vi "运维调试_五参数.vi"() -> ()   [LabVIEW 2016, in "斯坦道仪器.lvlib"]
uses:
  <vilib>/Utility/miscctls.llb/LVPointTypeDef.ctl
  PLC/PLC.lvlib
panel:
  in  "打开串口":bool
  in  "释放串口":bool
  in  "手动通电":bool
  out "多参数横条运行状态":T1(xcontrol)
  in  "数据区":i32(listbox)
  in  "探头选择":u16(ring)=9 items=["氨氮"=3, "水温"=9, "pH值"=10, "溶解氧"=11, "电导率"=12, "浊度"=13, "叶绿素a"=14, "藻密度"=15, "蓝绿藻"=16, "氧化还原电位"=17, "溶解氧%"=18, "盐度"=19]
  in  "测量数据区读取":bool
  in  "测量数据区":i32(listbox)
  in  "状态告警区读取":bool
  in  "状态告警区":i32(listbox)
  in  "自动校准":bool
  in  "读取KB":bool
  in  "写入KB":bool
  out "B":dbl caption="校准值B:"
  out "K":dbl caption="校准值K:"
  in  "校准区探头选择":u16(ring)=9 items=["氨氮"=3, "水温"=9, "pH值"=10, "溶解氧"=11, "电导率"=12, "浊度"=13, "叶绿素a"=14, "藻密度"=15, "蓝绿藻"=16, "氧化还原电位"=17, "溶解氧%"=18, "盐度"=19]
  in  "停止测量(单探)":bool
  in  "启动测量(单探)":bool
  in  "控制命令区探头选择":u16(ring)=9 items=["氨氮"=3, "水温"=9, "pH值"=10, "溶解氧"=11, "电导率"=12, "浊度"=13, "叶绿素a"=14, "藻密度"=15, "蓝绿藻"=16, "氧化还原电位"=17, "溶解氧%"=18, "盐度"=19]
  in  "同步时间":bool
  in  "初始化(清洗)":bool
  in  "停止测量(全部)":bool
  in  "启动测量(全部)":bool
  in  "关键参数区读取":bool
  in  "关键参数区":i32(listbox)
  in  "传感器参数读取":bool
  in  "传感器区":i32(listbox)
  in  "返回":bool
  in  "设置":bool
  out "运行状态":string
  out "开机状态":bool
  in  "停止":bool
  in  "手动启动":bool
  out "集成报警信息":string
  # "控制命令区"
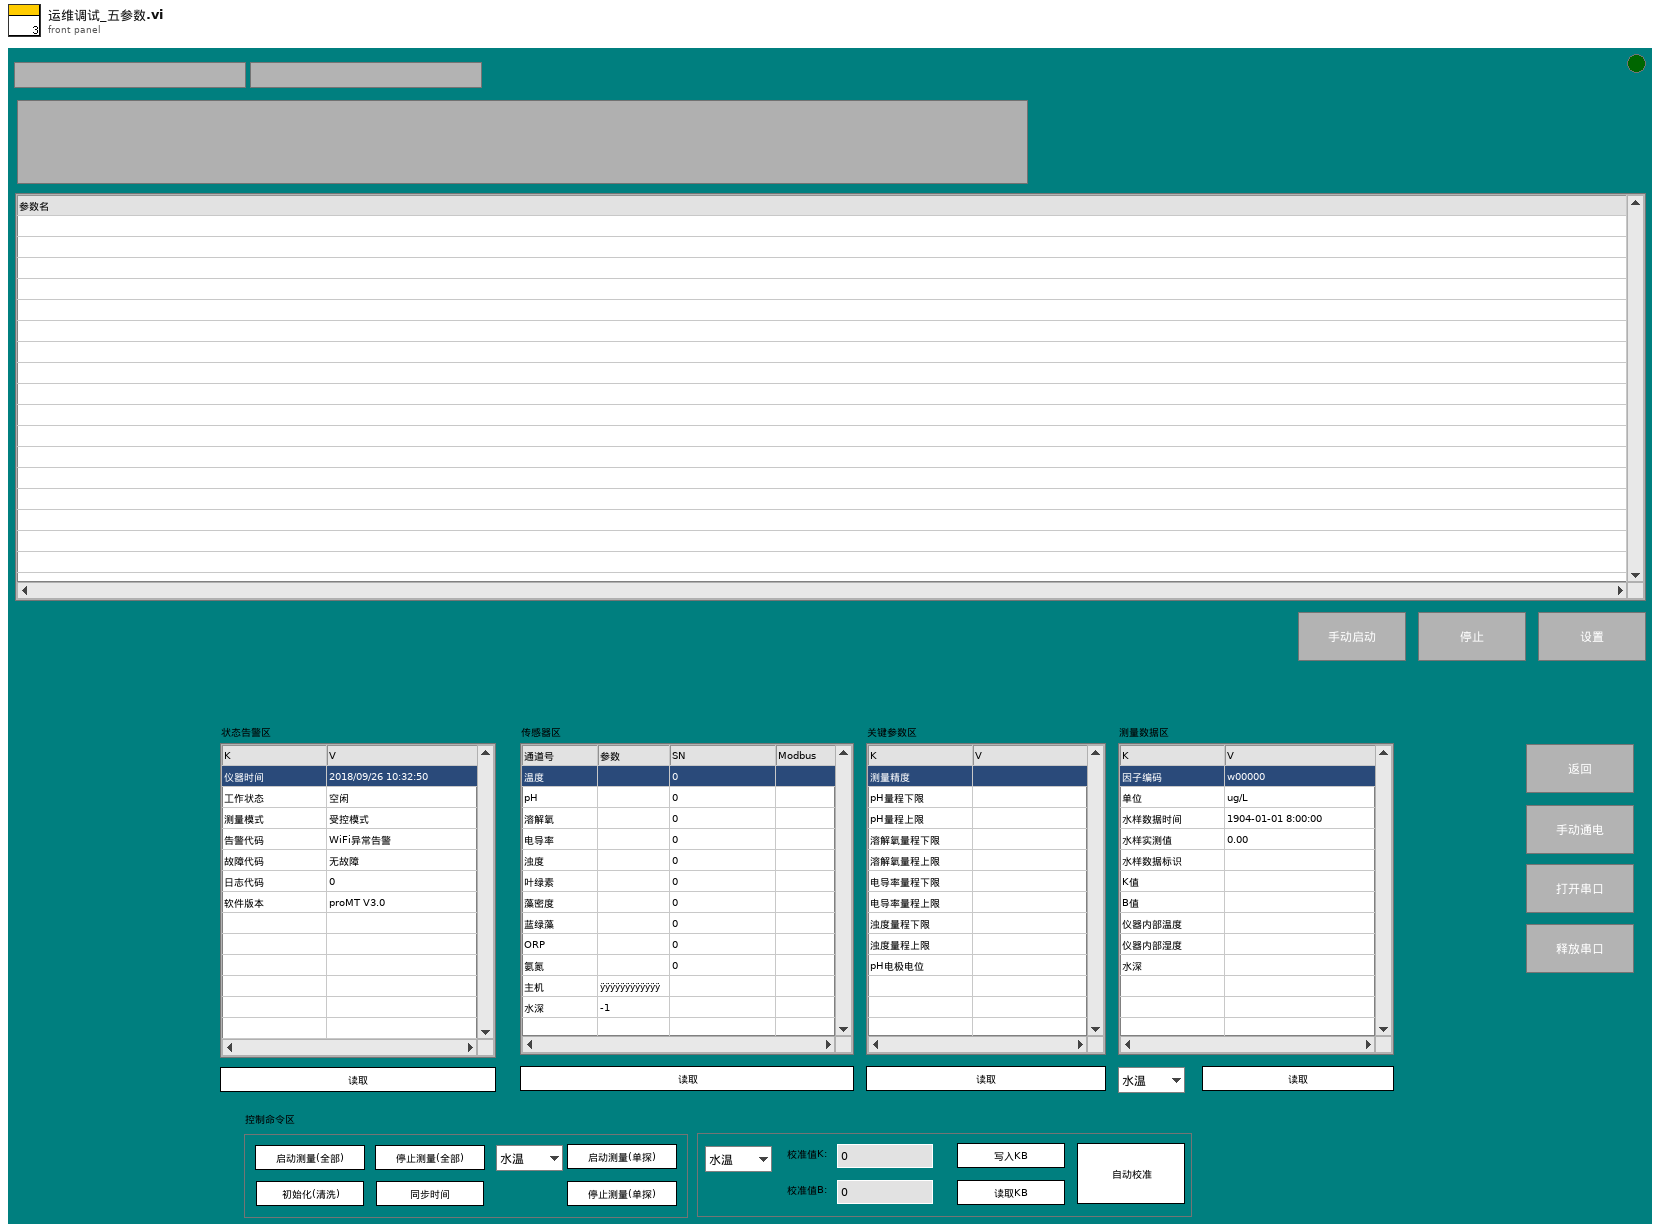
[diagram p1: front panel]
types:
  T1 = cluster{"系统时间":timestamp, "工作状态":u16, "测量模式":u16, "告警代码":enum16{"无告警", "缺试剂告警", "缺水样告警", "缺蒸馏水告警", "缺标液告警", "仪表漏液告警", "标定异常告警", "超量程告警", "加热异常", "低试剂预警", "超上限告警", "超下限告警", "仪表内部其他异常", "滴定异常告警", "电极异常告警", "量程切换告警", "参数设置告警", "PH电极电位异常", "电导率电极异常", "浊度光度异常", "溶解氧电极异常", "溶解氧光强异常", "温度异常告警", "PH异常告警", "溶解氧异常告警", "电导率异常告警", "浊度异常告警", "叶绿素异常告警", "藻密度异常告警", "蓝绿藻异常告警", "ORP异常告警", "氨氮异常告警", "清洁刷异常告警", "SD卡异常告警", "蓝牙异常告警", "Wifi异常告警", "流程异常告警"}, "故障代码":enum16{"无故障", "电机故障", "温度故障", "通讯故障", "滴定故障"}, "日志代码":u16, "软件版本":string}
  T2 = typedef "LVPointTypeDef.ctl" = cluster{"Horizontal":i16, "Vertical":i16}
  T3 = cluster{"时间标识":timestamp, "设备":string, "日志信息":string}
  T4 = enum16{"无告警", "缺试剂告警", "缺水样告警", "缺蒸馏水告警", "缺标液告警", "仪表漏液告警", "标定异常告警", "超量程告警", "加热异常", "低试剂预警", "超上限告警", "超下限告警", "仪表内部其他异常", "滴定异常告警", "电极异常告警", "量程切换告警", "参数设置告警", "PH电极电位异常", "电导率电极异常", "浊度光度异常", "溶解氧电极异常", "溶解氧光强异常", "温度异常告警", "PH异常告警", "溶解氧异常告警", "电导率异常告警", "浊度异常告警", "叶绿素异常告警", "藻密度异常告警", "蓝绿藻异常告警", "ORP异常告警", "氨氮异常告警", "清洁刷异常告警", "SD卡异常告警", "蓝牙异常告警", "Wifi异常告警", "流程异常告警"}
  T5 = cluster{"水温":dbl, "pH":dbl, "DO":dbl, "Cond":dbl, "Turb":dbl, "叶绿素":dbl, "藻密度":dbl, "蓝绿藻":dbl, "ORP":dbl, "NH3N":dbl}
  T6 = cluster{"因子编码":string, "单位":string, "标样参考值":sgl, "水样数据时间":timestamp, "水样实测值":sgl, "水样数据标识":string, "K":sgl, "B":sgl, "T":sgl, "H":sgl, "水深":sgl}
  T7 = enum8{"Enabled", "Disabled", "Disabled and Grayed Out"}
  T8 = cluster{"测量模式":enum16{"待机", "水样测试", "标样核查", "零点核查", "跨度核查", "空白测试", "平行样测试", "加标回收", "空白校准", "标样校准", "初始化（清洗）"}, "数据标记表":string, "测量时间":dbl}
  T9 = cluster{"starting address":u16, "holding register value":u16}
  T10 = enum16{"idle", "init", "读状态", "读参数", "多个写入", "单个写入", "线圈写入"}
  T11 = enum32{"Bad", "Idle", "Run top level", "Running"}
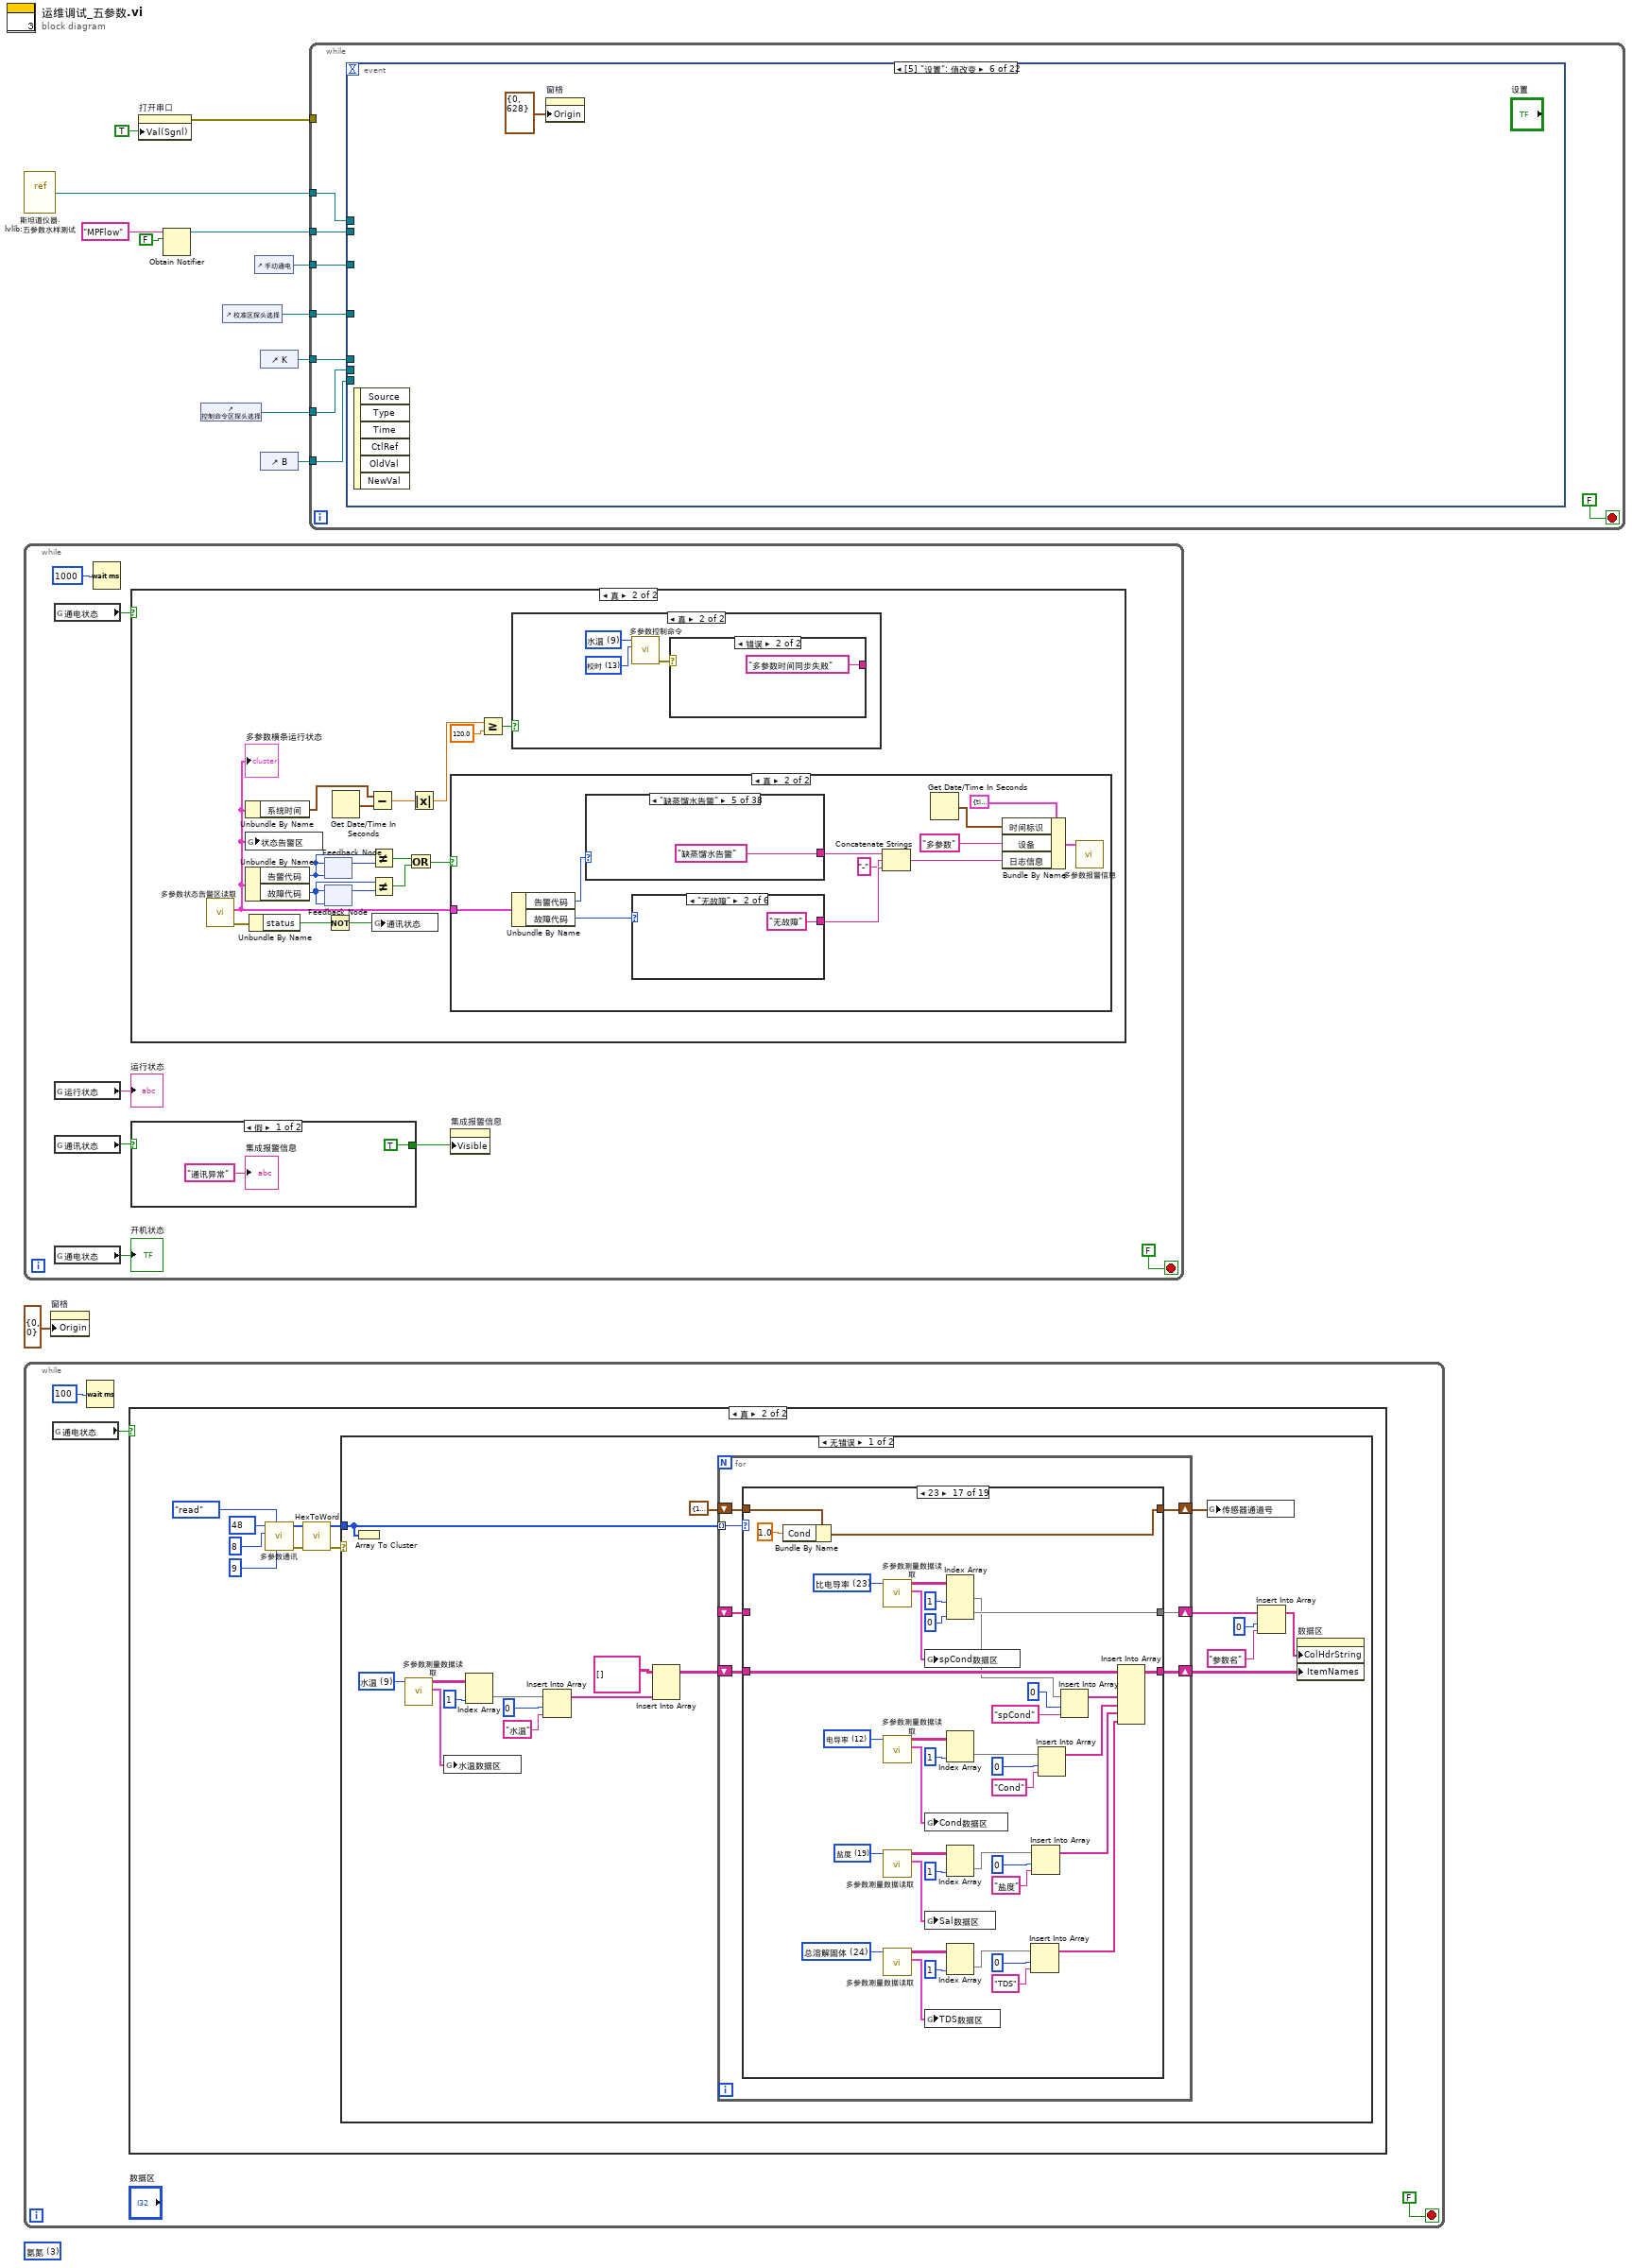
[diagram p0: block diagram]
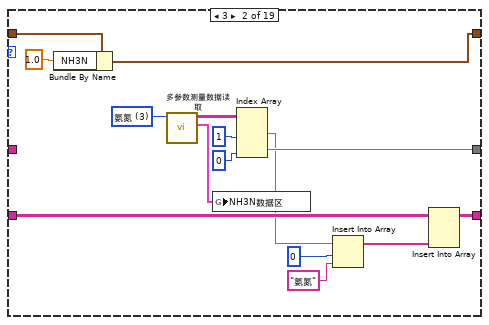
[diagram p4: hidden frame]
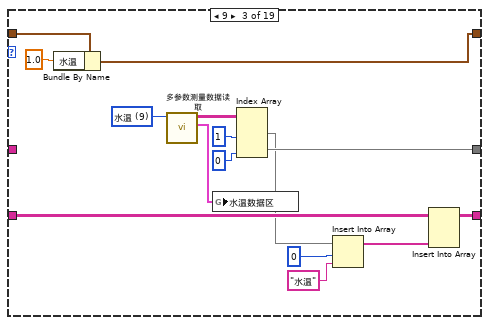
[diagram p5: hidden frame]
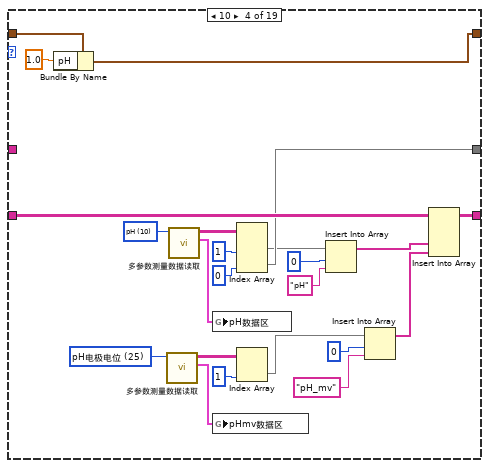
[diagram p6: hidden frame]
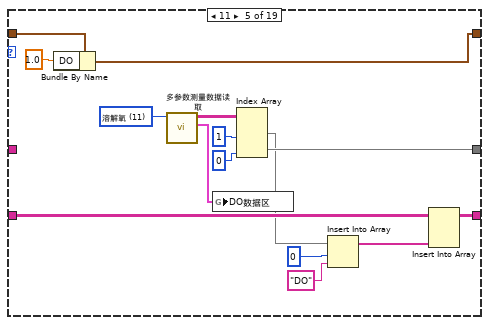
[diagram p7: hidden frame]
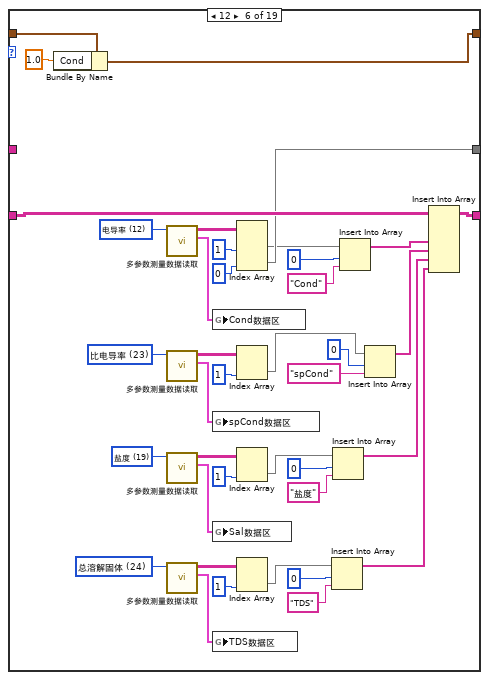
[diagram p8: hidden frame]
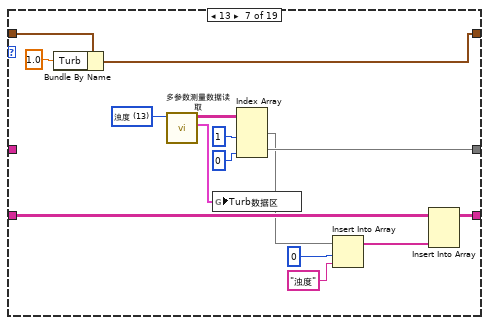
[diagram p9: hidden frame]
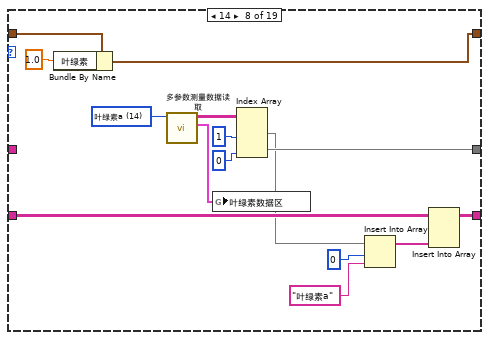
[diagram p10: hidden frame]
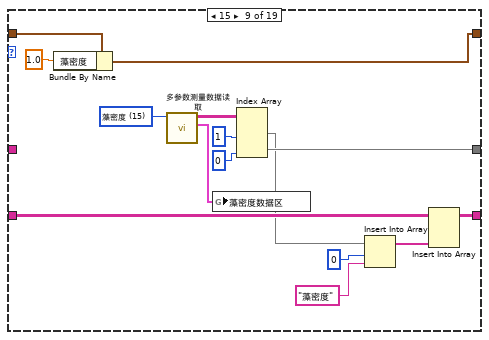
[diagram p11: hidden frame]
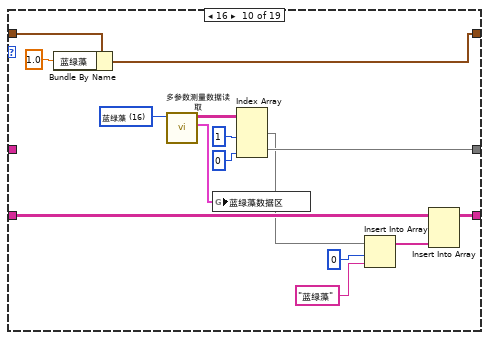
[diagram p12: hidden frame]
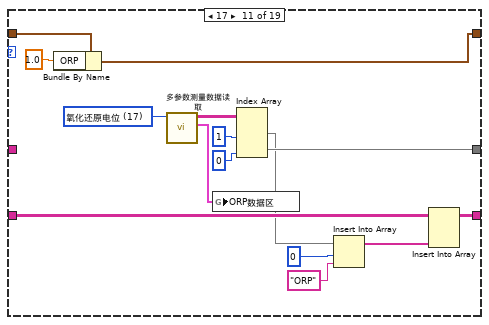
[diagram p13: hidden frame]
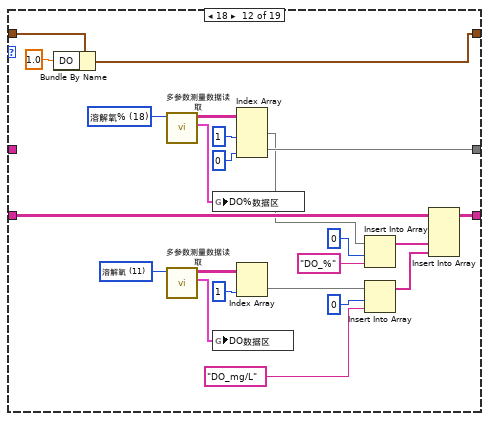
[diagram p14: hidden frame]
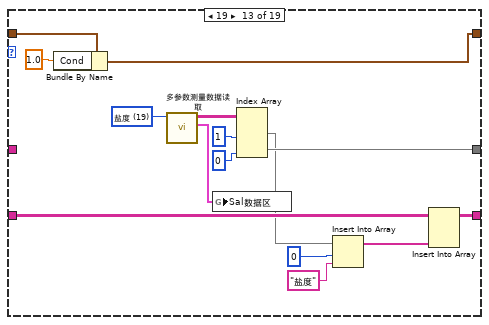
[diagram p15: hidden frame]
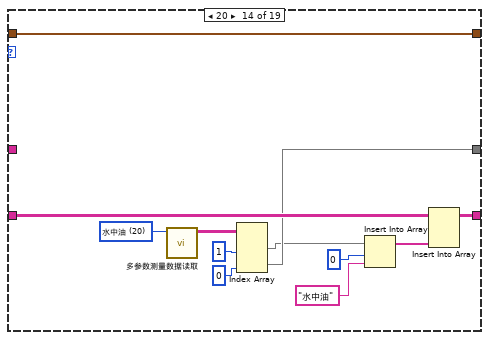
[diagram p16: hidden frame]
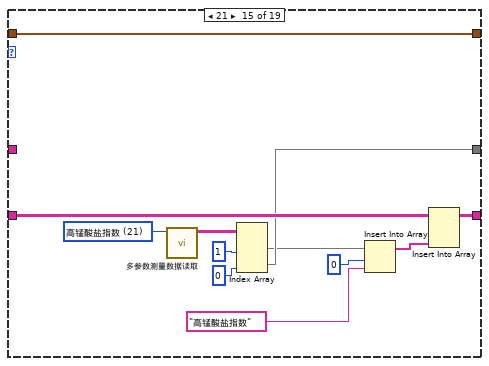
[diagram p17: hidden frame]
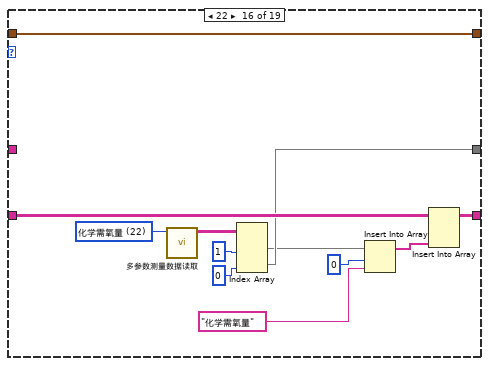
[diagram p18: hidden frame]
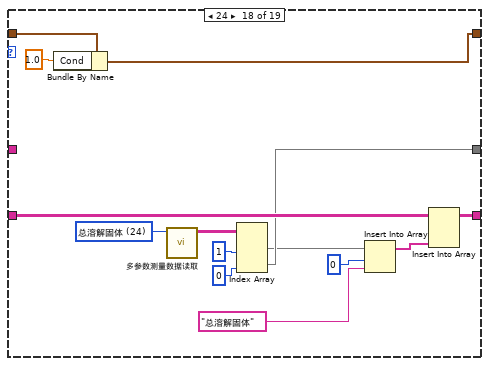
[diagram p19: hidden frame]
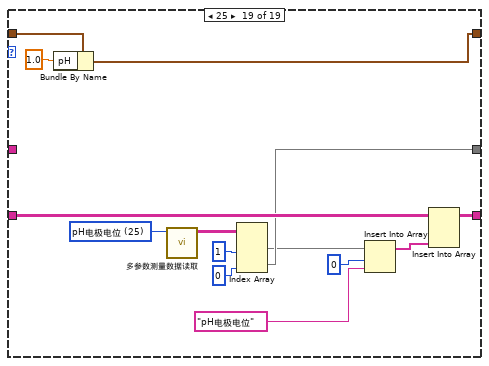
[diagram p20: hidden frame]
diagram:
  (unwired) u16 3 items=["氨氮"=3, "水温"=9, "pH"=10, "溶解氧"=11, "电导率"=12, "浊度"=13, "叶绿素a"=14, "藻密度"=15, "蓝绿藻"=16, "氧化还原电位"=17, "溶解氧%"=18, "盐度"=19, "水中油"=20, "高锰酸盐指数"=21, "化学需氧量"=22, "比电导率"=23, "总溶解固体"=24, "pH电极电位"=25] ("下拉列表")
  n1 = vi-ref "斯坦道仪器.lvlib:五参数水样测试.vi"() -> (w9:refnum<vi>)
  n2 = while {
    stop <- FALSE stop-if-true
    n3 = global read "多参数全局变量.vi" "通电状态"() -> (w13:bool)
    n4 = global read "多参数全局变量.vi" "运行状态"() -> (→"运行状态":string)
    n5 = global read "多参数全局变量.vi" "通讯状态"() -> (w17:bool)
    n6 = global read "多参数全局变量.vi" "通电状态"() -> (→"开机状态":bool)
    n7 = Wait (ms)(milliseconds to wait=u32 1000 ("等待时间（毫秒）")) -> ()  [unwired: 1 out]
    n8 = case shown="真" w13 {
      frame False {
      }
      frame True {
        n9 = call "多参数状态告警区读取.vi"() -> ("error out"=w29:errorcluster, "状态告警块"=w26:T1)  [unwired: 9 in, 1 out]
        "多参数横条运行状态" <- w26
        n10 = Unbundle By Name(w26) -> ("系统时间"=w25:timestamp)
        n11 = global write "多参数全局变量.vi" "状态告警区"(w26) -> ()
        n12 = Unbundle By Name(w26) -> ("告警代码"=w35:T4, "故障代码"=w33:enum16{"无故障", "电机故障", "温度故障", "通讯故障", "滴定故障"})
        n13 = Unbundle By Name(w29) -> ("status"=w28:bool)
        n14 = feedback #1(w35) -> (w36:T4)
        n15 = feedback-in #1(w35) -> ()
        n16 = feedback #2(w33) -> (w34:enum16{"无故障", "电机故障", "温度故障", "通讯故障", "滴定故障"})
        n17 = feedback-in #2(w33) -> ()
        n18 = Not(x=w28) -> (.not. x?=w27:bool)
        n19 = Get Date/Time In Seconds() -> (seconds since 1Jan1904=w24:timestamp)
        n20 = Subtract(x=w25, y=w24) -> (x-y=w23:dbl)
        n21 = Not Equal?(x=w35, y=w36) -> (x != y?=w31:bool)
        n22 = Not Equal?(x=w33, y=w34) -> (x != y?=w32:bool)
        n23 = global write "多参数全局变量.vi" "通讯状态"(w27) -> ()
        n24 = Or(x=w31, y=w32) -> (x .or. y?=w30:bool)
        n25 = Absolute Value(x=w23) -> (abs(x)=w22:dbl)
        n26 = case shown="真" w30 {
          tunnel: w26 -> [_ w52]
          frame False {
          }
          frame True {
            n27 = Unbundle By Name(w52) -> ("告警代码"=w51:T4, "故障代码"=w50:enum16{"无故障", "电机故障", "温度故障", "通讯故障", "滴定故障"})
            n28 = case shown="\"缺蒸馏水告警\"" w51 {
              selector: w51 -> [w63 _ _ _ _ _ _ _ _ _ _ _ _ _ _ _ _ _ _ _ _ _ _ _ _ _ _ _ _ _ _ _ _ _ _ _ _ _]
              tunnel: [w62 "无告警" "缺试剂告警" "缺水样告警" "缺蒸馏水告警" "缺标液告警" "仪表漏液告警" "标定异常告警" "超量程告警" "加热异常" "低试剂预警" "超上限告警" "超下限告警" "仪表内部其他异常" "滴定异常告警" "电极异常告警" "量程切换告警" "参数设置告警" "PH电极电位异常" "电导率电极异常" "浊度光度异常" "溶解氧电极异常" "溶解氧光强异常" "温度异常告警" "PH异常告警" "溶解氧异常告警" "电导率异常告警" "浊度异常告警" "叶绿素异常告警" "藻密度异常告警" "蓝绿藻异常告警" "ORP异常告警" "氨氮异常告警" "清洁刷异常告警" "SD卡异常告警" "蓝牙异常告警" "WiFi异常告警" "流程异常告警"] -> w49
              frame Default {
                n29 = Format Into String(format string="%d" ("格式字符串"), initial string="未知" ("工作状态"), w63) -> (resulting string=w62:string)  [unwired: 1 in, 1 out]
              }
              frame "无告警" {
              }
              frame "缺试剂告警" {
              }
              frame "缺水样告警" {
              }
              frame "缺蒸馏水告警" {
              }
              frame "缺标液告警" {
              }
              frame "仪表漏液告警" {
              }
              frame "标定异常告警" {
              }
              frame "超量程告警" {
              }
              frame "加热异常" {
              }
              frame "低试剂预警" {
              }
              frame "超上限告警" {
              }
              frame "超下限告警" {
              }
              frame "仪表内部其他异常" {
              }
              frame "滴定异常告警" {
              }
              frame "电极异常告警" {
              }
              frame "量程切换告警" {
              }
              frame "参数设置告警" {
              }
              frame "PH电极电位异常" {
              }
              frame "电导率电极异常" {
              }
              frame "浊度光度异常" {
              }
              frame "溶解氧电极异常" {
              }
              frame "溶解氧光强异常" {
              }
              frame "温度异常告警" {
              }
              frame "PH异常告警" {
              }
              frame "溶解氧异常告警" {
              }
              frame "电导率异常告警" {
              }
              frame "浊度异常告警" {
              }
              frame "叶绿素异常告警" {
              }
              frame "藻密度异常告警" {
              }
              frame "蓝绿藻异常告警" {
              }
              frame "ORP异常告警" {
              }
              frame "氨氮异常告警" {
              }
              frame "清洁刷异常告警" {
              }
              frame "SD卡异常告警" {
              }
              frame "蓝牙异常告警" {
              }
              frame "Wifi异常告警" {
              }
              frame "流程异常告警" {
              }
            }
            n30 = case shown="\"无故障\"" w50 {
              selector: w50 -> [w54 _ _ _ _ _]
              tunnel: [w53 "无故障" "电机故障" "温度故障" "通讯故障" "滴定故障"] -> w48
              frame Default {
                n31 = Format Into String(format string="%d" ("格式字符串"), initial string="未知" ("工作状态"), w54) -> (resulting string=w53:string)  [unwired: 1 in, 1 out]
              }
              frame "无故障" {
              }
              frame "电机故障" {
              }
              frame "温度故障" {
              }
              frame "通讯故障" {
              }
              frame "滴定故障" {
              }
            }
            n32 = Concatenate Strings(w49, "-" ("字符串"), w48) -> (w44:string)
            n33 = Get Date/Time In Seconds() -> (seconds since 1Jan1904=w43:timestamp)
            n34 = Bundle By Name(cluster=T3 {"时间标识"=timestamp(0 s since 1904-01-01), "设备"="", "日志信息"=""} ("data in"), "时间标识"=w43, "设备"="多参数", "日志信息"=w44) -> (w45:T3)
            n35 = call "多参数报警信息.vi"("data in"=w45) -> ()  [unwired: 10 in, 1 out]
          }
        }
        n36 = Greater Or Equal?(x=w22, y=120.0) -> (x >= y?=w21:bool)
        n37 = case shown="真" w21 {
          frame False {
          }
          frame True {
            w37 = u16 13 items=["启动测量（全部）"=1, "初始化（清洗）"=10, "停止测量（全部）"=11, "校时"=13, "启动测量（单个传感器）"=19, "停止测量（单个传感器）"=20] ("控制命令")
            w38 = u16 9 items=["氨氮"=3, "水温"=9, "pH值"=10, "溶解氧"=11, "电导率"=12, "浊度"=13, "叶绿素a"=14, "藻密度"=15, "蓝绿藻"=16, "氧化还原电位"=17, "溶解氧%"=18, "盐度"=19] ("站号")
            n38 = call "多参数控制命令.vi"("控制命令"=w37, "站号"=w38) -> ("error out"=w39:errorcluster)  [unwired: 9 in]
            n39 = case shown="错误" w39 {
              tunnel: ["多参数时间同步成功" ("消息") "多参数时间同步失败" ("消息")] -> _
              frame No Error {
              }
              frame Error {
              }
            }
          }
        }
      }
    }
    n40 = case shown="假" w17 {
      tunnel: [TRUE ("可见") _] -> w16
      frame False {
        "集成报警信息" <- "通讯异常" ("集成报警信息")
      }
      frame True {
      }
    }
    n41 = property on="集成报警信息" class="Str"("Visible"=w16) -> ()  [unwired: 2 in, 2 out]
  }
  n42 = while {
    stop <- FALSE stop-if-true
    n43 = global read "多参数全局变量.vi" "通电状态"() -> (w105:bool)
    n44 = Wait (ms)(milliseconds to wait=u32 100 ("等待时间（毫秒）")) -> ()  [unwired: 1 out]
    n45 = case shown="真" w105 {
      frame False {
      }
      frame True {
        n46 = call "多参数通讯.vi"("Slave ID"=u8 9, "STEP"=enum16{"open", "read", "write", "close"}."read", "quantity"=u16 8, "starting address"=u16 48) -> ("error out"=w110:errorcluster, "Registers"=w111:u16[])  [unwired: 5 in, 1 out]
        n47 = call "HexToWord.vi"("数组"=w111) -> ("WORD"=w114:u16[])  [unwired: 10 in]
        n48 = case shown="无错误" w110 {
          tunnel: w114 -> [w129 _]
          frame No Error {
            w126 = u16 9 items=["氨氮"=3, "水温"=9, "pH"=10, "溶解氧"=11, "电导率"=12, "浊度"=13, "叶绿素a"=14, "藻密度"=15, "蓝绿藻"=16, "氧化还原电位"=17, "溶解氧%"=18, "盐度"=19, "水中油"=20, "高锰酸盐指数"=21, "化学需氧量"=22, "比电导率"=23, "总溶解固体"=24, "pH电极电位"=25] ("下拉列表")
            n49 = Array To Cluster(array=w129) -> ()  [unwired: 1 out]
            n50 = call "多参数测量数据读取.vi"("探头选择"=w126) -> ("测量数据块"=w115:T6, "添加的数组"=w125:string[][])  [unwired: 8 in, 1 out]
            n51 = global write "多参数全局变量.vi" "水温数据区"(w115) -> ()
            n52 = Index Array(array=w125, index (col)=1 ("禁用的索引 (列)")) -> (element=w120:string[])  [unwired: 1 in]
            n53 = Insert Into Array(array=w120, index=0 ("索引"), new element="水温") -> (w122:string[])
            n54 = Insert Into Array(array=string[][] [] ("子数组"), new element=w122) -> (w118:string[][])  [unwired: 2 in]
            n55 = for {
              tunnel: w129 -> [w139] mode=indexing
              shift-right: [w137] -> w127
              shift-left: w118 -> [w138]
              shift-right: [w136] -> w128
              shift-left: _ -> [w135]
              shift-right: [w134] -> w116
              shift-left: T5 {"水温"=1.0, "pH"=0.0, "DO"=0.0, "Cond"=0.0, "Turb"=0.0, "叶绿素"=0.0, "藻密度"=0.0, "蓝绿藻"=0.0, "ORP"=0.0, "NH3N"=0.0} ("传感器通道号") -> [w133]
              n56 = case shown="23" w139 {
                tunnel: w138 -> [w142 w153 w168 w191 w206 w245 w260 w275 w290 w305 w320 w343 w358 w370 w382 w394 w433 w447 w461]
                tunnel: [w142 w152 w167 w190 w205 w244 w259 w274 w289 w304 w319 w342 w357 w369 w381 w393 w432 w446 w460] -> w137
                tunnel: [w141 w150 w165 w188 w203 w242 w257 w272 w287 w302 w317 w340 w355 w367 w379 w391 w430 w444 w458] -> w136
                tunnel: w135 -> [w141 _ _ _ _ _ _ _ _ _ _ _ _ _ _ _ _ _ _]
                tunnel: [w140 w144 w159 w175 w197 w215 w251 w266 w281 w296 w311 w327 w349 w363 w375 w387 w424 w438 w452] -> w134
                tunnel: w133 -> [w140 w146 w161 w177 w199 w216 w252 w267 w282 w297 w312 w328 w350 w363 w375 w387 w425 w439 w453]
                frame 0, Default {
                }
                frame 3 {
                  w157 = u16 3 items=["氨氮"=3, "水温"=9, "pH"=10, "溶解氧"=11, "电导率"=12, "浊度"=13, "叶绿素a"=14, "藻密度"=15, "蓝绿藻"=16, "氧化还原电位"=17, "溶解氧%"=18, "盐度"=19, "水中油"=20, "高锰酸盐指数"=21, "化学需氧量"=22, "比电导率"=23, "总溶解固体"=24, "pH电极电位"=25] ("下拉列表")
                  n57 = Bundle By Name(cluster=w146, "NH3N"=1.0) -> (w144:T5)
                  n58 = call "多参数测量数据读取.vi"("探头选择"=w157) -> ("测量数据块"=w143:T6, "添加的数组"=w156:string[][])  [unwired: 8 in, 1 out]
                  n59 = global write "多参数全局变量.vi" "NH3N数据区"(w143) -> ()
                  n60 = Index Array(array=w156, index (col) #1=1 ("禁用的索引 (列)"), index (col) #2=0 ("禁用的索引 (列)")) -> (element #1=w147:string[], element #2=w150:string[])  [unwired: 2 in]
                  n61 = Insert Into Array(array=w147, index=0 ("索引"), new element="氨氮") -> (w151:string[])
                  n62 = Insert Into Array(array=w153, new element=w151) -> (w152:string[][])  [unwired: 2 in]
                }
                frame 9 {
                  w172 = u16 9 items=["氨氮"=3, "水温"=9, "pH"=10, "溶解氧"=11, "电导率"=12, "浊度"=13, "叶绿素a"=14, "藻密度"=15, "蓝绿藻"=16, "氧化还原电位"=17, "溶解氧%"=18, "盐度"=19, "水中油"=20, "高锰酸盐指数"=21, "化学需氧量"=22, "比电导率"=23, "总溶解固体"=24, "pH电极电位"=25] ("下拉列表")
                  n63 = Bundle By Name(cluster=w161, "水温"=1.0) -> (w159:T5)
                  n64 = call "多参数测量数据读取.vi"("探头选择"=w172) -> ("测量数据块"=w158:T6, "添加的数组"=w171:string[][])  [unwired: 8 in, 1 out]
                  n65 = global write "多参数全局变量.vi" "水温数据区"(w158) -> ()
                  n66 = Index Array(array=w171, index (col) #1=1 ("禁用的索引 (列)"), index (col) #2=0 ("禁用的索引 (列)")) -> (element #1=w162:string[], element #2=w165:string[])  [unwired: 2 in]
                  n67 = Insert Into Array(array=w162, index=0 ("索引"), new element="水温") -> (w166:string[])
                  n68 = Insert Into Array(array=w168, new element=w166) -> (w167:string[][])  [unwired: 2 in]
                }
                frame 10 {
                  w179 = u16 25 items=["氨氮"=3, "水温"=9, "pH"=10, "溶解氧"=11, "电导率"=12, "浊度"=13, "叶绿素a"=14, "藻密度"=15, "蓝绿藻"=16, "氧化还原电位"=17, "溶解氧%"=18, "盐度"=19, "水中油"=20, "高锰酸盐指数"=21, "化学需氧量"=22, "比电导率"=23, "总溶解固体"=24, "pH电极电位"=25] ("下拉列表")
                  w195 = u16 10 items=["氨氮"=3, "水温"=9, "pH"=10, "溶解氧"=11, "电导率"=12, "浊度"=13, "叶绿素a"=14, "藻密度"=15, "蓝绿藻"=16, "氧化还原电位"=17, "溶解氧%"=18, "盐度"=19, "水中油"=20, "高锰酸盐指数"=21, "化学需氧量"=22, "比电导率"=23, "总溶解固体"=24, "pH电极电位"=25] ("下拉列表")
                  n69 = Bundle By Name(cluster=w177, "pH"=1.0) -> (w175:T5)
                  n70 = call "多参数测量数据读取.vi"("探头选择"=w179) -> ("测量数据块"=w173:T6, "添加的数组"=w180:string[][])  [unwired: 8 in, 1 out]
                  n71 = call "多参数测量数据读取.vi"("探头选择"=w195) -> ("测量数据块"=w174:T6, "添加的数组"=w194:string[][])  [unwired: 8 in, 1 out]
                  n72 = global write "多参数全局变量.vi" "pH数据区"(w174) -> ()
                  n73 = global write "多参数全局变量.vi" "pHmv数据区"(w173) -> ()
                  n74 = Index Array(array=w194, index (col) #1=1 ("禁用的索引 (列)"), index (col) #2=0 ("禁用的索引 (列)")) -> (element #1=w185:string[], element #2=w188:string[])  [unwired: 2 in]
                  n75 = Index Array(array=w180, index (col)=1 ("禁用的索引 (列)")) -> (element=w184:string[])  [unwired: 1 in]
                  n76 = Insert Into Array(array=w185, index=0 ("索引"), new element="pH") -> (w189:string[])
                  n77 = Insert Into Array(array=w184, index=0 ("索引"), new element="pH_mv") -> (w178:string[])
                  n78 = Insert Into Array(array=w191, new element #1=w189, new element #2=w178) -> (w190:string[][])  [unwired: 2 in]
                }
                frame 11 {
                  w210 = u16 11 items=["氨氮"=3, "水温"=9, "pH"=10, "溶解氧"=11, "电导率"=12, "浊度"=13, "叶绿素a"=14, "藻密度"=15, "蓝绿藻"=16, "氧化还原电位"=17, "溶解氧%"=18, "盐度"=19, "水中油"=20, "高锰酸盐指数"=21, "化学需氧量"=22, "比电导率"=23, "总溶解固体"=24, "pH电极电位"=25] ("下拉列表")
                  n79 = Bundle By Name(cluster=w199, "DO"=1.0) -> (w197:T5)
                  n80 = call "多参数测量数据读取.vi"("探头选择"=w210) -> ("测量数据块"=w196:T6, "添加的数组"=w209:string[][])  [unwired: 8 in, 1 out]
                  n81 = global write "多参数全局变量.vi" "DO数据区"(w196) -> ()
                  n82 = Index Array(array=w209, index (col) #1=1 ("禁用的索引 (列)"), index (col) #2=0 ("禁用的索引 (列)")) -> (element #1=w200:string[], element #2=w203:string[])  [unwired: 2 in]
                  n83 = Insert Into Array(array=w200, index=0 ("索引"), new element="DO") -> (w204:string[])
                  n84 = Insert Into Array(array=w206, new element=w204) -> (w205:string[][])  [unwired: 2 in]
                }
                frame 12 {
                  w219 = u16 24 items=["氨氮"=3, "水温"=9, "pH"=10, "溶解氧"=11, "电导率"=12, "浊度"=13, "叶绿素a"=14, "藻密度"=15, "蓝绿藻"=16, "氧化还原电位"=17, "溶解氧%"=18, "盐度"=19, "水中油"=20, "高锰酸盐指数"=21, "化学需氧量"=22, "比电导率"=23, "总溶解固体"=24, "pH电极电位"=25] ("下拉列表")
                  w231 = u16 19 items=["氨氮"=3, "水温"=9, "pH"=10, "溶解氧"=11, "电导率"=12, "浊度"=13, "叶绿素a"=14, "藻密度"=15, "蓝绿藻"=16, "氧化还原电位"=17, "溶解氧%"=18, "盐度"=19, "水中油"=20, "高锰酸盐指数"=21, "化学需氧量"=22, "比电导率"=23, "总溶解固体"=24, "pH电极电位"=25] ("下拉列表")
                  w233 = u16 23 items=["氨氮"=3, "水温"=9, "pH"=10, "溶解氧"=11, "电导率"=12, "浊度"=13, "叶绿素a"=14, "藻密度"=15, "蓝绿藻"=16, "氧化还原电位"=17, "溶解氧%"=18, "盐度"=19, "水中油"=20, "高锰酸盐指数"=21, "化学需氧量"=22, "比电导率"=23, "总溶解固体"=24, "pH电极电位"=25] ("下拉列表")
                  w249 = u16 12 items=["氨氮"=3, "水温"=9, "pH"=10, "溶解氧"=11, "电导率"=12, "浊度"=13, "叶绿素a"=14, "藻密度"=15, "蓝绿藻"=16, "氧化还原电位"=17, "溶解氧%"=18, "盐度"=19, "水中油"=20, "高锰酸盐指数"=21, "化学需氧量"=22, "比电导率"=23, "总溶解固体"=24, "pH电极电位"=25] ("下拉列表")
                  n85 = Bundle By Name(cluster=w216, "Cond"=1.0 ("DO")) -> (w215:T5)
                  n86 = call "多参数测量数据读取.vi"("探头选择"=w249) -> ("测量数据块"=w214:T6, "添加的数组"=w248:string[][])  [unwired: 8 in, 1 out]
                  n87 = call "多参数测量数据读取.vi"("探头选择"=w233) -> ("测量数据块"=w212:T6, "添加的数组"=w234:string[][])  [unwired: 8 in, 1 out]
                  n88 = call "多参数测量数据读取.vi"("探头选择"=w231) -> ("测量数据块"=w213:T6, "添加的数组"=w230:string[][])  [unwired: 8 in, 1 out]
                  n89 = call "多参数测量数据读取.vi"("探头选择"=w219) -> ("测量数据块"=w211:T6, "添加的数组"=w220:string[][])  [unwired: 8 in, 1 out]
                  n90 = global write "多参数全局变量.vi" "Cond数据区"(w214) -> ()
                  n91 = global write "多参数全局变量.vi" "spCond数据区"(w212) -> ()
                  n92 = global write "多参数全局变量.vi" "Sal数据区"(w213) -> ()
                  n93 = global write "多参数全局变量.vi" "TDS数据区"(w211) -> ()
                  n94 = Index Array(array=w248, index (col) #1=1 ("禁用的索引 (列)"), index (col) #2=0 ("禁用的索引 (列)")) -> (element #1=w239:string[], element #2=w242:string[])  [unwired: 2 in]
                  n95 = Index Array(array=w234, index (col)=1 ("禁用的索引 (列)")) -> (element=w238:string[])  [unwired: 1 in]
                  n96 = Index Array(array=w230, index (col)=1 ("禁用的索引 (列)")) -> (element=w226:string[])  [unwired: 1 in]
                  n97 = Index Array(array=w220, index (col)=1 ("禁用的索引 (列)")) -> (element=w224:string[])  [unwired: 1 in]
                  n98 = Insert Into Array(array=w224, index=0 ("索引"), new element="TDS") -> (w218:string[])
                  n99 = Insert Into Array(array=w226, index=0 ("索引"), new element="盐度") -> (w225:string[])
                  n100 = Insert Into Array(array=w239, index=0 ("索引"), new element="Cond") -> (w243:string[])
                  n101 = Insert Into Array(array=w238, index=0 ("索引"), new element="spCond") -> (w232:string[])
                  n102 = Insert Into Array(array=w245, new element #1=w243, new element #2=w232, new element #3=w225, new element #4=w218) -> (w244:string[][])  [unwired: 2 in]
                }
                frame 13 {
                  w264 = u16 13 items=["氨氮"=3, "水温"=9, "pH"=10, "溶解氧"=11, "电导率"=12, "浊度"=13, "叶绿素a"=14, "藻密度"=15, "蓝绿藻"=16, "氧化还原电位"=17, "溶解氧%"=18, "盐度"=19, "水中油"=20, "高锰酸盐指数"=21, "化学需氧量"=22, "比电导率"=23, "总溶解固体"=24, "pH电极电位"=25] ("下拉列表")
                  n103 = Bundle By Name(cluster=w252, "Turb"=1.0 ("DO")) -> (w251:T5)
                  n104 = call "多参数测量数据读取.vi"("探头选择"=w264) -> ("测量数据块"=w250:T6, "添加的数组"=w263:string[][])  [unwired: 8 in, 1 out]
                  n105 = global write "多参数全局变量.vi" "Turb数据区"(w250) -> ()
                  n106 = Index Array(array=w263, index (col) #1=1 ("禁用的索引 (列)"), index (col) #2=0 ("禁用的索引 (列)")) -> (element #1=w254:string[], element #2=w257:string[])  [unwired: 2 in]
                  n107 = Insert Into Array(array=w254, index=0 ("索引"), new element="浊度") -> (w258:string[])
                  n108 = Insert Into Array(array=w260, new element=w258) -> (w259:string[][])  [unwired: 2 in]
                }
                frame 14 {
                  w279 = u16 14 items=["氨氮"=3, "水温"=9, "pH"=10, "溶解氧"=11, "电导率"=12, "浊度"=13, "叶绿素a"=14, "藻密度"=15, "蓝绿藻"=16, "氧化还原电位"=17, "溶解氧%"=18, "盐度"=19, "水中油"=20, "高锰酸盐指数"=21, "化学需氧量"=22, "比电导率"=23, "总溶解固体"=24, "pH电极电位"=25] ("下拉列表")
                  n109 = Bundle By Name(cluster=w267, "叶绿素"=1.0 ("DO")) -> (w266:T5)
                  n110 = call "多参数测量数据读取.vi"("探头选择"=w279) -> ("测量数据块"=w265:T6, "添加的数组"=w278:string[][])  [unwired: 8 in, 1 out]
                  n111 = global write "多参数全局变量.vi" "叶绿素数据区"(w265) -> ()
                  n112 = Index Array(array=w278, index (col) #1=1 ("禁用的索引 (列)"), index (col) #2=0 ("禁用的索引 (列)")) -> (element #1=w269:string[], element #2=w272:string[])  [unwired: 2 in]
                  n113 = Insert Into Array(array=w269, index=0 ("索引"), new element="叶绿素a") -> (w273:string[])
                  n114 = Insert Into Array(array=w275, new element=w273) -> (w274:string[][])  [unwired: 2 in]
                }
                frame 15 {
                  w294 = u16 15 items=["氨氮"=3, "水温"=9, "pH"=10, "溶解氧"=11, "电导率"=12, "浊度"=13, "叶绿素a"=14, "藻密度"=15, "蓝绿藻"=16, "氧化还原电位"=17, "溶解氧%"=18, "盐度"=19, "水中油"=20, "高锰酸盐指数"=21, "化学需氧量"=22, "比电导率"=23, "总溶解固体"=24, "pH电极电位"=25] ("下拉列表")
                  n115 = Bundle By Name(cluster=w282, "藻密度"=1.0 ("DO")) -> (w281:T5)
                  n116 = call "多参数测量数据读取.vi"("探头选择"=w294) -> ("测量数据块"=w280:T6, "添加的数组"=w293:string[][])  [unwired: 8 in, 1 out]
                  n117 = global write "多参数全局变量.vi" "藻密度数据区"(w280) -> ()
                  n118 = Index Array(array=w293, index (col) #1=1 ("禁用的索引 (列)"), index (col) #2=0 ("禁用的索引 (列)")) -> (element #1=w284:string[], element #2=w287:string[])  [unwired: 2 in]
                  n119 = Insert Into Array(array=w284, index=0 ("索引"), new element="藻密度") -> (w288:string[])
                  n120 = Insert Into Array(array=w290, new element=w288) -> (w289:string[][])  [unwired: 2 in]
                }
                frame 16 {
                  w309 = u16 16 items=["氨氮"=3, "水温"=9, "pH"=10, "溶解氧"=11, "电导率"=12, "浊度"=13, "叶绿素a"=14, "藻密度"=15, "蓝绿藻"=16, "氧化还原电位"=17, "溶解氧%"=18, "盐度"=19, "水中油"=20, "高锰酸盐指数"=21, "化学需氧量"=22, "比电导率"=23, "总溶解固体"=24, "pH电极电位"=25] ("下拉列表")
                  n121 = Bundle By Name(cluster=w297, "蓝绿藻"=1.0 ("DO")) -> (w296:T5)
                  n122 = call "多参数测量数据读取.vi"("探头选择"=w309) -> ("测量数据块"=w295:T6, "添加的数组"=w308:string[][])  [unwired: 8 in, 1 out]
                  n123 = global write "多参数全局变量.vi" "蓝绿藻数据区"(w295) -> ()
                  n124 = Index Array(array=w308, index (col) #1=1 ("禁用的索引 (列)"), index (col) #2=0 ("禁用的索引 (列)")) -> (element #1=w299:string[], element #2=w302:string[])  [unwired: 2 in]
                  n125 = Insert Into Array(array=w299, index=0 ("索引"), new element="蓝绿藻") -> (w303:string[])
                  n126 = Insert Into Array(array=w305, new element=w303) -> (w304:string[][])  [unwired: 2 in]
                }
                frame 17 {
                  w324 = u16 17 items=["氨氮"=3, "水温"=9, "pH"=10, "溶解氧"=11, "电导率"=12, "浊度"=13, "叶绿素a"=14, "藻密度"=15, "蓝绿藻"=16, "氧化还原电位"=17, "溶解氧%"=18, "盐度"=19, "水中油"=20, "高锰酸盐指数"=21, "化学需氧量"=22, "比电导率"=23, "总溶解固体"=24, "pH电极电位"=25] ("下拉列表")
                  n127 = Bundle By Name(cluster=w312, "ORP"=1.0 ("DO")) -> (w311:T5)
                  n128 = call "多参数测量数据读取.vi"("探头选择"=w324) -> ("测量数据块"=w310:T6, "添加的数组"=w323:string[][])  [unwired: 8 in, 1 out]
                  n129 = global write "多参数全局变量.vi" "ORP数据区"(w310) -> ()
                  n130 = Index Array(array=w323, index (col) #1=1 ("禁用的索引 (列)"), index (col) #2=0 ("禁用的索引 (列)")) -> (element #1=w314:string[], element #2=w317:string[])  [unwired: 2 in]
                  n131 = Insert Into Array(array=w314, index=0 ("索引"), new element="ORP") -> (w318:string[])
                  n132 = Insert Into Array(array=w320, new element=w318) -> (w319:string[][])  [unwired: 2 in]
                }
                frame 18 {
                  w331 = u16 11 items=["氨氮"=3, "水温"=9, "pH"=10, "溶解氧"=11, "电导率"=12, "浊度"=13, "叶绿素a"=14, "藻密度"=15, "蓝绿藻"=16, "氧化还原电位"=17, "溶解氧%"=18, "盐度"=19, "水中油"=20, "高锰酸盐指数"=21, "化学需氧量"=22, "比电导率"=23, "总溶解固体"=24, "pH电极电位"=25] ("下拉列表")
                  w347 = u16 18 items=["氨氮"=3, "水温"=9, "pH"=10, "溶解氧"=11, "电导率"=12, "浊度"=13, "叶绿素a"=14, "藻密度"=15, "蓝绿藻"=16, "氧化还原电位"=17, "溶解氧%"=18, "盐度"=19, "水中油"=20, "高锰酸盐指数"=21, "化学需氧量"=22, "比电导率"=23, "总溶解固体"=24, "pH电极电位"=25] ("下拉列表")
                  n133 = Bundle By Name(cluster=w328, "DO"=1.0) -> (w327:T5)
                  n134 = call "多参数测量数据读取.vi"("探头选择"=w347) -> ("测量数据块"=w326:T6, "添加的数组"=w346:string[][])  [unwired: 8 in, 1 out]
                  n135 = call "多参数测量数据读取.vi"("探头选择"=w331) -> ("测量数据块"=w325:T6, "添加的数组"=w332:string[][])  [unwired: 8 in, 1 out]
                  n136 = global write "多参数全局变量.vi" "DO%数据区"(w326) -> ()
                  n137 = global write "多参数全局变量.vi" "DO数据区"(w325) -> ()
                  n138 = Index Array(array=w346, index (col) #1=1 ("禁用的索引 (列)"), index (col) #2=0 ("禁用的索引 (列)")) -> (element #1=w337:string[], element #2=w340:string[])  [unwired: 2 in]
                  n139 = Index Array(array=w332, index (col)=1 ("禁用的索引 (列)")) -> (element=w336:string[])  [unwired: 1 in]
                  n140 = Insert Into Array(array=w337, index=0 ("索引"), new element="DO_%") -> (w341:string[])
                  n141 = Insert Into Array(array=w336, index=0 ("索引"), new element="DO_mg/L") -> (w330:string[])
                  n142 = Insert Into Array(array=w343, new element #1=w341, new element #2=w330) -> (w342:string[][])  [unwired: 2 in]
                }
                frame 19 {
                  w362 = u16 19 items=["氨氮"=3, "水温"=9, "pH"=10, "溶解氧"=11, "电导率"=12, "浊度"=13, "叶绿素a"=14, "藻密度"=15, "蓝绿藻"=16, "氧化还原电位"=17, "溶解氧%"=18, "盐度"=19, "水中油"=20, "高锰酸盐指数"=21, "化学需氧量"=22, "比电导率"=23, "总溶解固体"=24, "pH电极电位"=25] ("下拉列表")
                  n143 = Bundle By Name(cluster=w350, "Cond"=1.0 ("DO")) -> (w349:T5)
                  n144 = call "多参数测量数据读取.vi"("探头选择"=w362) -> ("测量数据块"=w348:T6, "添加的数组"=w361:string[][])  [unwired: 8 in, 1 out]
                  n145 = global write "多参数全局变量.vi" "Sal数据区"(w348) -> ()
                  n146 = Index Array(array=w361, index (col) #1=1 ("禁用的索引 (列)"), index (col) #2=0 ("禁用的索引 (列)")) -> (element #1=w352:string[], element #2=w355:string[])  [unwired: 2 in]
                  n147 = Insert Into Array(array=w352, index=0 ("索引"), new element="盐度") -> (w356:string[])
                  n148 = Insert Into Array(array=w358, new element=w356) -> (w357:string[][])  [unwired: 2 in]
                }
                frame 20 {
                  w374 = u16 20 items=["氨氮"=3, "水温"=9, "pH"=10, "溶解氧"=11, "电导率"=12, "浊度"=13, "叶绿素a"=14, "藻密度"=15, "蓝绿藻"=16, "氧化还原电位"=17, "溶解氧%"=18, "盐度"=19, "水中油"=20, "高锰酸盐指数"=21, "化学需氧量"=22, "比电导率"=23, "总溶解固体"=24, "pH电极电位"=25] ("下拉列表")
                  n149 = call "多参数测量数据读取.vi"("探头选择"=w374) -> ("添加的数组"=w373:string[][])  [unwired: 8 in, 2 out]
                  n150 = Index Array(array=w373, index (col) #1=1 ("禁用的索引 (列)"), index (col) #2=0 ("禁用的索引 (列)")) -> (element #1=w364:string[], element #2=w367:string[])  [unwired: 2 in]
                  n151 = Insert Into Array(array=w364, index=0 ("索引"), new element="水中油") -> (w368:string[])
                  n152 = Insert Into Array(array=w370, new element=w368) -> (w369:string[][])  [unwired: 2 in]
                }
                frame 21 {
                  w386 = u16 21 items=["氨氮"=3, "水温"=9, "pH"=10, "溶解氧"=11, "电导率"=12, "浊度"=13, "叶绿素a"=14, "藻密度"=15, "蓝绿藻"=16, "氧化还原电位"=17, "溶解氧%"=18, "盐度"=19, "水中油"=20, "高锰酸盐指数"=21, "化学需氧量"=22, "比电导率"=23, "总溶解固体"=24, "pH电极电位"=25] ("下拉列表")
                  n153 = call "多参数测量数据读取.vi"("探头选择"=w386) -> ("添加的数组"=w385:string[][])  [unwired: 8 in, 2 out]
                  n154 = Index Array(array=w385, index (col) #1=1 ("禁用的索引 (列)"), index (col) #2=0 ("禁用的索引 (列)")) -> (element #1=w376:string[], element #2=w379:string[])  [unwired: 2 in]
                  n155 = Insert Into Array(array=w376, index=0 ("索引"), new element="高锰酸盐指数") -> (w380:string[])
                  n156 = Insert Into Array(array=w382, new element=w380) -> (w381:string[][])  [unwired: 2 in]
                }
                frame 22 {
                  w398 = u16 22 items=["氨氮"=3, "水温"=9, "pH"=10, "溶解氧"=11, "电导率"=12, "浊度"=13, "叶绿素a"=14, "藻密度"=15, "蓝绿藻"=16, "氧化还原电位"=17, "溶解氧%"=18, "盐度"=19, "水中油"=20, "高锰酸盐指数"=21, "化学需氧量"=22, "比电导率"=23, "总溶解固体"=24, "pH电极电位"=25] ("下拉列表")
                  n157 = call "多参数测量数据读取.vi"("探头选择"=w398) -> ("添加的数组"=w397:string[][])  [unwired: 8 in, 2 out]
                  n158 = Index Array(array=w397, index (col) #1=1 ("禁用的索引 (列)"), index (col) #2=0 ("禁用的索引 (列)")) -> (element #1=w388:string[], element #2=w391:string[])  [unwired: 2 in]
                  n159 = Insert Into Array(array=w388, index=0 ("索引"), new element="化学需氧量") -> (w392:string[])
                  n160 = Insert Into Array(array=w394, new element=w392) -> (w393:string[][])  [unwired: 2 in]
                }
                frame 23 {
                  w406 = u16 24 items=["氨氮"=3, "水温"=9, "pH"=10, "溶解氧"=11, "电导率"=12, "浊度"=13, "叶绿素a"=14, "藻密度"=15, "蓝绿藻"=16, "氧化还原电位"=17, "溶解氧%"=18, "盐度"=19, "水中油"=20, "高锰酸盐指数"=21, "化学需氧量"=22, "比电导率"=23, "总溶解固体"=24, "pH电极电位"=25] ("下拉列表")
                  w417 = u16 19 items=["氨氮"=3, "水温"=9, "pH"=10, "溶解氧"=11, "电导率"=12, "浊度"=13, "叶绿素a"=14, "藻密度"=15, "蓝绿藻"=16, "氧化还原电位"=17, "溶解氧%"=18, "盐度"=19, "水中油"=20, "高锰酸盐指数"=21, "化学需氧量"=22, "比电导率"=23, "总溶解固体"=24, "pH电极电位"=25] ("下拉列表")
                  w418 = u16 12 items=["氨氮"=3, "水温"=9, "pH"=10, "溶解氧"=11, "电导率"=12, "浊度"=13, "叶绿素a"=14, "藻密度"=15, "蓝绿藻"=16, "氧化还原电位"=17, "溶解氧%"=18, "盐度"=19, "水中油"=20, "高锰酸盐指数"=21, "化学需氧量"=22, "比电导率"=23, "总溶解固体"=24, "pH电极电位"=25] ("下拉列表")
                  w437 = u16 23 items=["氨氮"=3, "水温"=9, "pH"=10, "溶解氧"=11, "电导率"=12, "浊度"=13, "叶绿素a"=14, "藻密度"=15, "蓝绿藻"=16, "氧化还原电位"=17, "溶解氧%"=18, "盐度"=19, "水中油"=20, "高锰酸盐指数"=21, "化学需氧量"=22, "比电导率"=23, "总溶解固体"=24, "pH电极电位"=25] ("下拉列表")
                  n161 = Bundle By Name(cluster=w425, "Cond"=1.0 ("DO")) -> (w424:T5)
                  n162 = call "多参数测量数据读取.vi"("探头选择"=w437) -> ("测量数据块"=w400:T6, "添加的数组"=w436:string[][])  [unwired: 8 in, 1 out]
                  n163 = call "多参数测量数据读取.vi"("探头选择"=w418) -> ("测量数据块"=w402:T6, "添加的数组"=w419:string[][])  [unwired: 8 in, 1 out]
                  n164 = call "多参数测量数据读取.vi"("探头选择"=w417) -> ("测量数据块"=w401:T6, "添加的数组"=w416:string[][])  [unwired: 8 in, 1 out]
                  n165 = call "多参数测量数据读取.vi"("探头选择"=w406) -> ("测量数据块"=w399:T6, "添加的数组"=w407:string[][])  [unwired: 8 in, 1 out]
                  n166 = global write "多参数全局变量.vi" "spCond数据区"(w400) -> ()
                  n167 = global write "多参数全局变量.vi" "Cond数据区"(w402) -> ()
                  n168 = global write "多参数全局变量.vi" "Sal数据区"(w401) -> ()
                  n169 = global write "多参数全局变量.vi" "TDS数据区"(w399) -> ()
                  n170 = Index Array(array=w436, index (col) #1=1 ("禁用的索引 (列)"), index (col) #2=0 ("禁用的索引 (列)")) -> (element #1=w427:string[], element #2=w430:string[])  [unwired: 2 in]
                  n171 = Index Array(array=w419, index (col)=1 ("禁用的索引 (列)")) -> (element=w423:string[])  [unwired: 1 in]
                  n172 = Index Array(array=w416, index (col)=1 ("禁用的索引 (列)")) -> (element=w412:string[])  [unwired: 1 in]
                  n173 = Index Array(array=w407, index (col)=1 ("禁用的索引 (列)")) -> (element=w411:string[])  [unwired: 1 in]
                  n174 = Insert Into Array(array=w411, index=0 ("索引"), new element="TDS") -> (w403:string[])
                  n175 = Insert Into Array(array=w412, index=0 ("索引"), new element="盐度") -> (w404:string[])
                  n176 = Insert Into Array(array=w423, index=0 ("索引"), new element="Cond") -> (w405:string[])
                  n177 = Insert Into Array(array=w427, index=0 ("索引"), new element="spCond") -> (w431:string[])
                  n178 = Insert Into Array(array=w433, new element #1=w431, new element #2=w405, new element #3=w404, new element #4=w403) -> (w432:string[][])  [unwired: 2 in]
                }
                frame 24 {
                  w451 = u16 24 items=["氨氮"=3, "水温"=9, "pH"=10, "溶解氧"=11, "电导率"=12, "浊度"=13, "叶绿素a"=14, "藻密度"=15, "蓝绿藻"=16, "氧化还原电位"=17, "溶解氧%"=18, "盐度"=19, "水中油"=20, "高锰酸盐指数"=21, "化学需氧量"=22, "比电导率"=23, "总溶解固体"=24, "pH电极电位"=25] ("下拉列表")
                  n179 = Bundle By Name(cluster=w439, "Cond"=1.0 ("DO")) -> (w438:T5)
                  n180 = call "多参数测量数据读取.vi"("探头选择"=w451) -> ("添加的数组"=w450:string[][])  [unwired: 8 in, 2 out]
                  n181 = Index Array(array=w450, index (col) #1=1 ("禁用的索引 (列)"), index (col) #2=0 ("禁用的索引 (列)")) -> (element #1=w441:string[], element #2=w444:string[])  [unwired: 2 in]
                  n182 = Insert Into Array(array=w441, index=0 ("索引"), new element="总溶解固体") -> (w445:string[])
                  n183 = Insert Into Array(array=w447, new element=w445) -> (w446:string[][])  [unwired: 2 in]
                }
                frame 25 {
                  w465 = u16 25 items=["氨氮"=3, "水温"=9, "pH"=10, "溶解氧"=11, "电导率"=12, "浊度"=13, "叶绿素a"=14, "藻密度"=15, "蓝绿藻"=16, "氧化还原电位"=17, "溶解氧%"=18, "盐度"=19, "水中油"=20, "高锰酸盐指数"=21, "化学需氧量"=22, "比电导率"=23, "总溶解固体"=24, "pH电极电位"=25] ("下拉列表")
                  n184 = Bundle By Name(cluster=w453, "pH"=1.0 ("DO")) -> (w452:T5)
                  n185 = call "多参数测量数据读取.vi"("探头选择"=w465) -> ("添加的数组"=w464:string[][])  [unwired: 8 in, 2 out]
                  n186 = Index Array(array=w464, index (col) #1=1 ("禁用的索引 (列)"), index (col) #2=0 ("禁用的索引 (列)")) -> (element #1=w455:string[], element #2=w458:string[])  [unwired: 2 in]
                  n187 = Insert Into Array(array=w455, index=0 ("索引"), new element="pH电极电位") -> (w459:string[])
                  n188 = Insert Into Array(array=w461, new element=w459) -> (w460:string[][])  [unwired: 2 in]
                }
              }
            }
            n189 = global write "多参数全局变量.vi" "传感器通道号"(w116) -> ()
            n190 = Insert Into Array(array=w128, index=0 ("索引"), new element="参数名" ("新元素/子数组")) -> (w132:string[])
            n191 = property on="数据区" class="MCListbox (严格)"("ColHdrString"=w132, "ItemNames"=w127) -> ()  [unwired: 2 in, 2 out]
          }
          frame Error {
          }
        }
      }
    }
  }
  n192 = property on="窗格" class="Pane"("Origin"=T2 {"Horizontal"=0, "Vertical"=0} ("原点")) -> ()  [unwired: 2 in, 2 out]
  n193 = property on="打开串口" class="Bool (严格)"("Val(Sgnl)"=TRUE ("值(信号)")) -> (error out=w1:errorcluster)  [unwired: 2 in, 1 out]
  n194 = Obtain Notifier(name (unnamed)="MPFlow" ("名称（未命名）"), notification data type=FALSE) -> (notifier out=w8:refnum<notifier>)  [unwired: 2 in, 2 out]
  n195 = control-ref of="控制命令区探头选择"() -> (w7:refnum<vi>)
  n196 = control-ref of="校准区探头选择"() -> (w4:refnum<vi>)
  n197 = control-ref of="手动通电"() -> (w3:refnum<vi>)
  n198 = control-ref of="K"() -> (w6:refnum<vi>)
  n199 = control-ref of="B"() -> (w5:refnum<vi>)
  n200 = while {
    tunnel: w9 -> [w472]
    tunnel: w8 -> [w471]
    tunnel: w7 -> [w470]
    tunnel: w6 -> [w469]
    tunnel: w5 -> [w468]
    tunnel: w4 -> [w467]
    tunnel: w3 -> [w466]
    tunnel: w1 -> [_]
    stop <- FALSE stop-if-true
    n201 = event shown="[5] \"设置\": 值改变" {
      selector: _ -> [_ _ _ _ _ _ _ _ _ _ _ _ _ _ _ _ _ _ _ _ _ _]
      dyn-events: _ -> [_ _ _ _ _ _ _ _ _ _ _ _ _ _ _ _ _ _ _ _ _ _]
      timeout: _ -> [_ _ _ _ _ _ _ _ _ _ _ _ _ _ _ _ _ _ _ _ _ _]
      tunnel: w472 -> [_ _ _ w488 _ _ _ _ _ _ _ _ _ _ _ _ _ _ _ _ _ _]
      tunnel: w471 -> [_ _ _ _ w510 _ _ _ _ _ _ _ _ _ _ _ _ _ _ _ _ _]
      tunnel: w470 -> [_ _ _ _ _ _ _ _ _ _ _ _ _ _ _ w577 w588 _ _ _ _ _]
      tunnel: w469 -> [_ _ _ _ _ _ _ _ _ _ _ _ _ _ _ _ _ w599 _ _ _ _]
      tunnel: w468 -> [_ _ _ _ _ _ _ _ _ _ _ _ _ _ _ _ _ w601 _ _ _ _]
      tunnel: w467 -> [_ _ _ _ _ _ _ _ _ _ _ _ _ _ _ _ _ w603 _ w619 _ _]
      tunnel: w466 -> [_ _ _ _ _ _ _ w518 w523 w528 w534 w539 w548 w557 w566 w575 w586 w597 _ w617 w629 _]
      event Timeout {
        n202 = event-data() -> ()  [unwired: 1 in, 3 out]
      }
      event "释放串口": Value Change {
        n203 = event-data() -> ("NewVal"=w474:bool)  [unwired: 1 in, 5 out]
        n204 = case shown="真" w474 {
          frame False {
          }
          frame True {
            n205 = call "多参数通讯.vi"("STEP"=enum16{"open", "read", "write", "close"}."close") -> ("error out"=w475:errorcluster)  [unwired: 8 in, 2 out]
            n206 = case shown="无错误" w475 {
              frame No Error {
                n207 = property on="打开串口" class="Bool (严格)"("DisabledEnum"=T7."Enabled" ("禁用")) -> ()  [unwired: 2 in, 2 out]
              }
              frame Error {
              }
            }
          }
        }
      }
      event "打开串口": Value Change {
        n208 = event-data() -> ("NewVal"=w478:bool)  [unwired: 1 in, 5 out]
        n209 = case shown="真" w478 {
          frame False {
          }
          frame True {
            n210 = call "多参数通讯.vi"("STEP"=enum16{"open", "read", "write", "close"}."open") -> ("error out"=w479:errorcluster)  [unwired: 8 in, 2 out]
            n211 = case shown="错误" w479 {
              tunnel: [T7."Disabled and Grayed Out" ("禁用") T7."Enabled" ("禁用")] -> w481
              frame No Error {
              }
              frame Error {
                n212 = One Button Dialog(message="多参数串口打开失败" ("消息")) -> ()  [unwired: 1 in, 1 out]
              }
            }
            n213 = property on="打开串口" class="Bool (严格)"("DisabledEnum"=w481, "Value"=FALSE ("打开串口")) -> ()  [unwired: 2 in, 2 out]
          }
        }
      }
      event "手动启动": Value Change {
        n214 = event-data() -> ()  [unwired: 1 in, 6 out]
        n215 = call "多参数启动参数对话框.vi"() -> ("确认"=w487:bool, "测量时间"=w486:dbl)  [unwired: 10 in]
        n216 = case shown="真" w487 {
          tunnel: w488 -> [_ w490]
          tunnel: w486 -> [_ w489]
          frame False {
          }
          frame True {
            n217 = property class="VI"(reference=w490) -> ("Name"=w494:string, "Exec.State"=w492:T11)  [unwired: 1 in, 2 out]
            n218 = Open VI Reference(type specifier VI Refnum (for type only)=refnum<vi> refnum ("类型说明符VI引用句柄（仅用于类型）"), vi path=w494, options=128 ("选项")) -> (vi reference=w493:refnum<vi>)  [unwired: 3 in, 1 out]
            n219 = case shown="\"Idle\"" w492 {
              tunnel: w493 -> [w498 w505]
              tunnel: [w498 w504] -> w491
              tunnel: w489 -> [_ w499]
              frame "Bad", Default {
                n220 = One Button Dialog(message="仪器已经启动，无需重复启动" ("消息")) -> ()  [unwired: 1 in, 1 out]
              }
              frame "Idle" {
                n221 = global read "系统变量.vi" "运行模式"() -> (w501:enum16{"维护模式", "常规模式", "应急模式", "质控模式"})
                n222 = case shown="\"常规模式\", 默认" w501 {
                  tunnel: ["M" ("数据标记表") "hd" ("数据标记表")] -> w500
                  frame "维护模式" {
                  }
                  frame "常规模式", Default {
                  }
                }
                n223 = Bundle By Name(cluster=T8 {"测量模式"=enum."水样测试", "数据标记表"="", "测量时间"=0.0} ("启动参数"), "数据标记表"=w500, "测量时间"=w499) -> (w502:T8)
                n224 = call-by-ref "开始异步调用"(reference=w505, "启动参数"=w502) -> (reference out=w504:refnum<vi>)  [unwired: 12 in, 1 out]
              }
            }
            n225 = Close Reference(reference=w491) -> ()  [unwired: 1 in, 1 out]
          }
        }
      }
      event "停止": Value Change {
        n226 = event-data() -> ()  [unwired: 1 in, 6 out]
        n227 = Two Button Dialog(message="请再一次确认是否停止测量" ("消息")) -> (T button?=w508:bool)  [unwired: 2 in]
        n228 = case shown="真" w508 {
          tunnel: w510 -> [_ w513]
          frame False {
          }
          frame True {
            w511 = u16 11 items=["启动测量（全部）"=1, "初始化（清洗）"=10, "停止测量（全部）"=11, "校时"=13, "启动测量（单个传感器）"=19, "停止测量（单个传感器）"=20] ("控制命令")
            w512 = u16 10 items=["氨氮"=3, "水温"=9, "pH值"=10, "溶解氧"=11, "电导率"=12, "浊度"=13, "叶绿素a"=14, "藻密度"=15, "蓝绿藻"=16, "氧化还原电位"=17, "溶解氧%"=18, "盐度"=19] ("站号")
            n229 = Send Notification(notification=TRUE ("通知"), notifier=w513) -> ()  [unwired: 1 in, 2 out]
            n230 = call "多参数控制命令.vi"("控制命令"=w511, "站号"=w512) -> ()  [unwired: 9 in, 1 out]
          }
        }
      }
      event "设置": Value Change {
        n231 = event-data() -> ()  [unwired: 1 in, 6 out]
        n232 = property on="窗格" class="Pane"("Origin"=T2 {"Horizontal"=0, "Vertical"=628} ("原点")) -> ()  [unwired: 2 in, 2 out]
      }
      event "返回": Value Change {
        n233 = event-data() -> ()  [unwired: 1 in, 6 out]
        n234 = property on="窗格" class="Pane"("Origin"=T2 {"Horizontal"=0, "Vertical"=0} ("原点")) -> ()  [unwired: 2 in, 2 out]
      }
      event "传感器参数读取": Value Change {
        n235 = event-data() -> ()  [unwired: 1 in, 6 out]
        n236 = property class="Bool (严格)"(reference=w518) -> ("Value"=w517:bool)  [unwired: 1 in, 2 out]
        n237 = case shown="真" w517 {
          frame False {
            n238 = One Button Dialog(message="启动失败，请先通电" ("消息")) -> ()  [unwired: 1 in, 1 out]
          }
          frame True {
            n239 = call "多参数传感器参数读取.vi"() -> ("error out"=w520:errorcluster, "添加的数组"=w521:string[][])  [unwired: 10 in]
            n240 = call <vilib>:"General Error Handler.vi"("error in (no error)"=w520) -> ()  [unwired: 10 in, 5 out]
            n241 = property on="传感器区" class="MCListbox (严格)"("ItemNames"=w521) -> ()  [unwired: 2 in, 2 out]
          }
        }
      }
      event "关键参数区读取": Value Change {
        n242 = event-data() -> ()  [unwired: 1 in, 6 out]
        n243 = property class="Bool (严格)"(reference=w523) -> ("Value"=w522:bool)  [unwired: 1 in, 2 out]
        n244 = case shown="假" w522 {
          frame False {
            n245 = One Button Dialog(message="启动失败，请先通电" ("消息")) -> ()  [unwired: 1 in, 1 out]
          }
          frame True {
            n246 = call "多参数关键参数读取.vi"() -> ("error out"=w525:errorcluster, "添加的数组"=w526:string[][])  [unwired: 10 in]
            n247 = call <vilib>:"General Error Handler.vi"("error in (no error)"=w525) -> ()  [unwired: 10 in, 5 out]
            n248 = property on="关键参数区" class="MCListbox (严格)"("ItemNames"=w526) -> ()  [unwired: 2 in, 2 out]
          }
        }
      }
      event "测量数据区读取": Value Change {
        n249 = event-data() -> ()  [unwired: 1 in, 6 out]
        n250 = property class="Bool (严格)"(reference=w528) -> ("Value"=w527:bool)  [unwired: 1 in, 2 out]
        n251 = case shown="假" w527 {
          frame False {
            n252 = One Button Dialog(message="启动失败，请先通电" ("消息")) -> ()  [unwired: 1 in, 1 out]
          }
          frame True {
            n253 = call "多参数测量数据读取.vi"("探头选择"="探头选择") -> ("error out"=w531:errorcluster, "添加的数组"=w532:string[][])  [unwired: 8 in, 1 out]
            n254 = call <vilib>:"General Error Handler.vi"("error in (no error)"=w531) -> ()  [unwired: 10 in, 5 out]
            n255 = property on="测量数据区" class="MCListbox (严格)"("ItemNames"=w532) -> ()  [unwired: 2 in, 2 out]
          }
        }
      }
      event "状态告警区读取": Value Change {
        n256 = event-data() -> ()  [unwired: 1 in, 6 out]
        n257 = property class="Bool (严格)"(reference=w534) -> ("Value"=w533:bool)  [unwired: 1 in, 2 out]
        n258 = case shown="真" w533 {
          frame False {
            n259 = One Button Dialog(message="启动失败，请先通电" ("消息")) -> ()  [unwired: 1 in, 1 out]
          }
          frame True {
            n260 = call "多参数状态告警区读取.vi"() -> ("error out"=w536:errorcluster, "添加的数组"=w537:string[][])  [unwired: 9 in, 1 out]
            n261 = call <vilib>:"General Error Handler.vi"("error in (no error)"=w536) -> ()  [unwired: 10 in, 5 out]
            n262 = property on="状态告警区" class="MCListbox (严格)"("ItemNames"=w537) -> ()  [unwired: 2 in, 2 out]
          }
        }
      }
      event "同步时间": Value Change {
        n263 = event-data() -> ()  [unwired: 1 in, 6 out]
        n264 = property class="Bool (严格)"(reference=w539) -> ("Value"=w538:bool)  [unwired: 1 in, 2 out]
        n265 = case shown="假" w538 {
          frame False {
            n266 = One Button Dialog(message="启动失败，请先通电" ("消息")) -> ()  [unwired: 1 in, 1 out]
          }
          frame True {
            w541 = u16 13 items=["启动测量（全部）"=1, "初始化（清洗）"=10, "停止测量（全部）"=11, "校时"=13, "启动测量（单个传感器）"=19, "停止测量（单个传感器）"=20] ("控制命令")
            w542 = u16 9 items=["氨氮"=3, "水温"=9, "pH值"=10, "溶解氧"=11, "电导率"=12, "浊度"=13, "叶绿素a"=14, "藻密度"=15, "蓝绿藻"=16, "氧化还原电位"=17, "溶解氧%"=18, "盐度"=19] ("站号")
            n267 = call "多参数控制命令.vi"("控制命令"=w541, "站号"=w542) -> ("error out"=w544:errorcluster)  [unwired: 9 in]
            n268 = case shown="错误" w544 {
              tunnel: ["时间同步成功" ("消息") "时间同步失败" ("消息")] -> w543
              frame No Error {
              }
              frame Error {
              }
            }
            n269 = One Button Dialog(message=w543) -> ()  [unwired: 1 in, 1 out]
          }
        }
      }
      event "启动测量(全部)": Value Change {
        n270 = event-data() -> ()  [unwired: 1 in, 6 out]
        n271 = property class="Bool (严格)"(reference=w548) -> ("Value"=w547:bool)  [unwired: 1 in, 2 out]
        n272 = case shown="假" w547 {
          frame False {
            n273 = One Button Dialog(message="启动失败，请先通电" ("消息")) -> ()  [unwired: 1 in, 1 out]
          }
          frame True {
            w550 = u16 1 items=["启动测量（全部）"=1, "初始化（清洗）"=10, "停止测量（全部）"=11, "校时"=13, "启动测量（单个传感器）"=19, "停止测量（单个传感器）"=20] ("控制命令")
            w551 = u16 9 items=["氨氮"=3, "水温"=9, "pH值"=10, "溶解氧"=11, "电导率"=12, "浊度"=13, "叶绿素a"=14, "藻密度"=15, "蓝绿藻"=16, "氧化还原电位"=17, "溶解氧%"=18, "盐度"=19] ("站号")
            n274 = call "多参数控制命令.vi"("控制命令"=w550, "站号"=w551) -> ("error out"=w553:errorcluster)  [unwired: 9 in]
            n275 = case shown="无错误" w553 {
              tunnel: ["启动成功" ("消息") "启动失败" ("消息")] -> w552
              frame No Error {
              }
              frame Error {
              }
            }
            n276 = One Button Dialog(message=w552) -> ()  [unwired: 1 in, 1 out]
          }
        }
      }
      event "停止测量(全部)": Value Change {
        n277 = event-data() -> ()  [unwired: 1 in, 6 out]
        n278 = property class="Bool (严格)"(reference=w557) -> ("Value"=w556:bool)  [unwired: 1 in, 2 out]
        n279 = case shown="真" w556 {
          frame False {
            n280 = One Button Dialog(message="启动失败，请先通电" ("消息")) -> ()  [unwired: 1 in, 1 out]
          }
          frame True {
            w561 = u16 11 items=["启动测量（全部）"=1, "初始化（清洗）"=10, "停止测量（全部）"=11, "校时"=13, "启动测量（单个传感器）"=19, "停止测量（单个传感器）"=20] ("控制命令")
            w562 = u16 9 items=["氨氮"=3, "水温"=9, "pH值"=10, "溶解氧"=11, "电导率"=12, "浊度"=13, "叶绿素a"=14, "藻密度"=15, "蓝绿藻"=16, "氧化还原电位"=17, "溶解氧%"=18, "盐度"=19] ("站号")
            n281 = call "多参数控制命令.vi"("控制命令"=w561, "站号"=w562) -> ("error out"=w560:errorcluster)  [unwired: 9 in]
            n282 = case shown="错误" w560 {
              tunnel: ["停止成功" ("消息") "停止失败" ("消息")] -> w559
              frame No Error {
              }
              frame Error {
              }
            }
            n283 = One Button Dialog(message=w559) -> ()  [unwired: 1 in, 1 out]
          }
        }
      }
      event "初始化(清洗)": Value Change {
        n284 = event-data() -> ()  [unwired: 1 in, 6 out]
        n285 = property class="Bool (严格)"(reference=w566) -> ("Value"=w565:bool)  [unwired: 1 in, 2 out]
        n286 = case shown="真" w565 {
          frame False {
            n287 = One Button Dialog(message="启动失败，请先通电" ("消息")) -> ()  [unwired: 1 in, 1 out]
          }
          frame True {
            w570 = u16 10 items=["启动测量（全部）"=1, "初始化（清洗）"=10, "停止测量（全部）"=11, "校时"=13, "启动测量（单个传感器）"=19, "停止测量（单个传感器）"=20] ("控制命令")
            w571 = u16 9 items=["氨氮"=3, "水温"=9, "pH值"=10, "溶解氧"=11, "电导率"=12, "浊度"=13, "叶绿素a"=14, "藻密度"=15, "蓝绿藻"=16, "氧化还原电位"=17, "溶解氧%"=18, "盐度"=19] ("站号")
            n288 = call "多参数控制命令.vi"("控制命令"=w570, "站号"=w571) -> ("error out"=w568:errorcluster)  [unwired: 9 in]
            n289 = case shown="错误" w568 {
              tunnel: ["初始化成功" ("消息") "初始化失败" ("消息")] -> w569
              frame No Error {
              }
              frame Error {
              }
            }
            n290 = One Button Dialog(message=w569) -> ()  [unwired: 1 in, 1 out]
          }
        }
      }
      event "启动测量(单探)": Value Change {
        n291 = event-data() -> ()  [unwired: 1 in, 6 out]
        n292 = property class="Bool (严格)"(reference=w575) -> ("Value"=w574:bool)  [unwired: 1 in, 2 out]
        n293 = property class="Ring (严格)"(reference=w577) -> ("Value"=w576:u16)  [unwired: 1 in, 2 out]
        n294 = case shown="真" w574 {
          tunnel: w576 -> [_ w579]
          frame False {
            n295 = One Button Dialog(message="启动失败，请先通电" ("消息")) -> ()  [unwired: 1 in, 1 out]
          }
          frame True {
            w580 = u16 19 items=["启动测量（全部）"=1, "初始化（清洗）"=10, "停止测量（全部）"=11, "校时"=13, "启动测量（单个传感器）"=19, "停止测量（单个传感器）"=20] ("控制命令")
            n296 = call "多参数控制命令.vi"("控制命令"=w580, "站号"=w579) -> ("error out"=w582:errorcluster)  [unwired: 9 in]
            n297 = case shown="无错误" w582 {
              tunnel: ["启动成功" ("消息") "启动失败" ("消息")] -> w581
              frame No Error {
              }
              frame Error {
              }
            }
            n298 = One Button Dialog(message=w581) -> ()  [unwired: 1 in, 1 out]
          }
        }
      }
      event "停止测量(单探)": Value Change {
        n299 = event-data() -> ()  [unwired: 1 in, 6 out]
        n300 = property class="Bool (严格)"(reference=w586) -> ("Value"=w585:bool)  [unwired: 1 in, 2 out]
        n301 = property class="Ring (严格)"(reference=w588) -> ("Value"=w587:u16)  [unwired: 1 in, 2 out]
        n302 = case shown="真" w585 {
          tunnel: w587 -> [_ w590]
          frame False {
            n303 = One Button Dialog(message="启动失败，请先通电" ("消息")) -> ()  [unwired: 1 in, 1 out]
          }
          frame True {
            w591 = u16 20 items=["启动测量（全部）"=1, "初始化（清洗）"=10, "停止测量（全部）"=11, "校时"=13, "启动测量（单个传感器）"=19, "停止测量（单个传感器）"=20] ("控制命令")
            n304 = call "多参数控制命令.vi"("控制命令"=w591, "站号"=w590) -> ("error out"=w593:errorcluster)  [unwired: 9 in]
            n305 = case shown="错误" w593 {
              tunnel: ["停止成功" ("消息") "停止失败" ("消息")] -> w592
              frame No Error {
              }
              frame Error {
              }
            }
            n306 = One Button Dialog(message=w592) -> ()  [unwired: 1 in, 1 out]
          }
        }
      }
      event "写入KB": Value Change {
        n307 = event-data() -> ()  [unwired: 1 in, 6 out]
        n308 = property class="DigNum (严格)"(reference=w599) -> ("Value"=w598:dbl)  [unwired: 1 in, 2 out]
        n309 = property class="DigNum (严格)"(reference=w601) -> ("Value"=w600:dbl)  [unwired: 1 in, 2 out]
        n310 = property class="Bool (严格)"(reference=w597) -> ("Value"=w596:bool)  [unwired: 1 in, 2 out]
        n311 = property class="Ring (严格)"(reference=w603) -> ("Value"=w602:u16)  [unwired: 1 in, 2 out]
        n312 = case shown="假" w596 {
          tunnel: w602 -> [_ w609]
          tunnel: w600 -> [_ w608]
          tunnel: w598 -> [_ w607]
          frame False {
            n313 = One Button Dialog(message="启动失败，请先通电" ("消息")) -> ()  [unwired: 1 in, 1 out]
          }
          frame True {
            n314 = call "多参数校准写入.vi"("B"=w608, "K"=w607, "站号"=w609) -> ("error out"=w605:errorcluster)  [unwired: 8 in]
            n315 = case shown="错误" w605 {
              tunnel: ["写入成功" ("消息") "写入失败" ("消息")] -> w606
              frame No Error {
              }
              frame Error {
              }
            }
            n316 = One Button Dialog(message=w606) -> ()  [unwired: 1 in, 1 out]
          }
        }
      }
      event "K", "B": Mouse Down {
        n317 = event-data() -> ("CtlRef"=w615:refnum<vi>)  [unwired: 1 in, 5 out]
        n318 = property class="DigNum (严格)"(reference=w615) -> (reference out=w614:refnum<vi>, "Value"=w613:dbl)  [unwired: 1 in, 1 out]
        n319 = call "数字键盘.vi"("OldNumber"=w613) -> ("NewNumber"=w612:sgl)
        n320 = property class="DigNum (严格)"(reference=w614, "Value"=w612) -> ()  [unwired: 1 in, 2 out]
      }
      event "读取KB": Value Change {
        n321 = event-data() -> ()  [unwired: 1 in, 6 out]
        n322 = property class="Bool (严格)"(reference=w617) -> ("Value"=w616:bool)  [unwired: 1 in, 2 out]
        n323 = property class="Ring (严格)"(reference=w619) -> ("Value"=w618:u16)  [unwired: 1 in, 2 out]
        n324 = case shown="真" w616 {
          tunnel: w618 -> [_ w623]
          frame False {
            n325 = One Button Dialog(message="启动失败，请先通电" ("消息")) -> ()  [unwired: 1 in, 1 out]
          }
          frame True {
            n326 = call "多参校准读取.vi"("站号"=w623) -> ("error out"=w621:errorcluster, "B"=→"B":dbl, "K"=→"K":dbl)  [unwired: 8 in]
            n327 = case shown="无错误" w621 {
              tunnel: ["读取成功" ("消息") "读取失败" ("消息")] -> w622
              frame No Error {
              }
              frame Error {
              }
            }
            n328 = One Button Dialog(message=w622) -> ()  [unwired: 1 in, 1 out]
          }
        }
      }
      event "自动校准": Value Change {
        n329 = event-data() -> ()  [unwired: 1 in, 6 out]
        n330 = property class="Bool (严格)"(reference=w629) -> ("Value"=w628:bool)  [unwired: 1 in, 2 out]
        n331 = case shown="真" w628 {
          frame False {
            n332 = One Button Dialog(message="启动失败，请先通电" ("消息")) -> ()  [unwired: 1 in, 1 out]
          }
          frame True {
            n333 = call "多参校准.vi"() -> ()  [unwired: 12 in]
          }
        }
      }
      event "手动通电": Value Change {
        n334 = event-data() -> ("NewVal"=w632:bool)  [unwired: 1 in, 5 out]
        n335 = Boolean To (0,1)(Boolean=w632) -> (0, 1=w631:i16)
        n336 = Bundle By Name(cluster=T9 {"starting address"=0, "holding register value"=0}, "starting address"=u16 302, "holding register value"=w631) -> (w634:T9)
        n337 = call "采配水通讯指令.vi"("数据"=w634, "命令"=T10."单个写入") -> ()  [unwired: 10 in]
      }
    }
  }
